vi "AlarmasGlobal.vi"() -> ()   [LabVIEW 2018]
uses:
  Controls/Cluster_Alarmas_IEEE45.ctl
  <vilib>/RAFA Solutions/Harmony UI Controls Kit/Boolean/Round Led.ctl
  <vilib>/RAFA Solutions/Harmony UI Controls Kit/Flat UI Design.lvlib
panel:
  out "G06_Alarmas_IEEE45":T1={"V1_V2 (V) "={0.0, 17.0, 16.662651515468255}, "Mod_V1_V2"=0.0, "alarma 1"=FALSE, "Mod_V2_V3"=0.0, "alarma 2"=FALSE, "Mod_V3_V1"=0.0, "alarma 3"=FALSE, "Mod_Frec"=0.0, "alarma 4"=FALSE, "V2_V3 (V)"={0.0, 17.0, 16.662651515468255}, "V3_V1 (V)"={0.0, 17.0, 16.662651515468255}, "Frecuencia (Hz)"={0.0, 17.0, 16.662651515468255}, "AVG VL_VL (V)"={0.0, 17.0, 16.662651515468255}, "alarm 5"=FALSE, "alarm 6"=FALSE, "alarm 7"=FALSE, "alarm 8"=FALSE, "alarm 9"=FALSE} {"AVG VL_VL (V)" scale=427.0..473.0; "Frecuencia (Hz)" scale=58.0..62.0; "V3_V1 (V)" scale=418.0..482.0; "V2_V3 (V)" scale=418.0..482.0; "Mod_Frec" format="%#.1f"; "Mod_V3_V1" format="%#.1f"; "Mod_V2_V3" format="%#.1f"; "Mod_V1_V2" format="%#.1f"; "V1_V2 (V)" scale=418.0..482.0}
  out "G05_Alarmas_IEEE45":T1={"V1_V2 (V) "={0.0, 17.0, 16.662651515468255}, "Mod_V1_V2"=0.0, "alarma 1"=FALSE, "Mod_V2_V3"=0.0, "alarma 2"=FALSE, "Mod_V3_V1"=0.0, "alarma 3"=FALSE, "Mod_Frec"=0.0, "alarma 4"=FALSE, "V2_V3 (V)"={0.0, 17.0, 16.662651515468255}, "V3_V1 (V)"={0.0, 17.0, 16.662651515468255}, "Frecuencia (Hz)"={0.0, 17.0, 16.662651515468255}, "AVG VL_VL (V)"={0.0, 17.0, 16.662651515468255}, "alarm 5"=FALSE, "alarm 6"=FALSE, "alarm 7"=FALSE, "alarm 8"=FALSE, "alarm 9"=FALSE} {"AVG VL_VL (V)" scale=427.0..473.0; "Frecuencia (Hz)" scale=58.0..62.0; "V3_V1 (V)" scale=418.0..482.0; "V2_V3 (V)" scale=418.0..482.0; "Mod_Frec" format="%#.1f"; "Mod_V3_V1" format="%#.1f"; "Mod_V2_V3" format="%#.1f"; "Mod_V1_V2" format="%#.1f"; "V1_V2 (V)" scale=418.0..482.0}
  out "G04_Alarmas_IEEE45":T1={"V1_V2 (V) "={0.0, 17.0, 16.662651515468255}, "Mod_V1_V2"=0.0, "alarma 1"=FALSE, "Mod_V2_V3"=0.0, "alarma 2"=FALSE, "Mod_V3_V1"=0.0, "alarma 3"=FALSE, "Mod_Frec"=0.0, "alarma 4"=FALSE, "V2_V3 (V)"={0.0, 17.0, 16.662651515468255}, "V3_V1 (V)"={0.0, 17.0, 16.662651515468255}, "Frecuencia (Hz)"={0.0, 17.0, 16.662651515468255}, "AVG VL_VL (V)"={0.0, 17.0, 16.662651515468255}, "alarm 5"=FALSE, "alarm 6"=FALSE, "alarm 7"=FALSE, "alarm 8"=FALSE, "alarm 9"=FALSE} {"AVG VL_VL (V)" scale=427.0..473.0; "Frecuencia (Hz)" scale=58.0..62.0; "V3_V1 (V)" scale=418.0..482.0; "V2_V3 (V)" scale=418.0..482.0; "Mod_Frec" format="%#.1f"; "Mod_V3_V1" format="%#.1f"; "Mod_V2_V3" format="%#.1f"; "Mod_V1_V2" format="%#.1f"; "V1_V2 (V)" scale=418.0..482.0}
  out "G03_Alarmas_IEEE45":T1={"V1_V2 (V) "={0.0, 17.0, 16.662651515468255}, "Mod_V1_V2"=0.0, "alarma 1"=FALSE, "Mod_V2_V3"=0.0, "alarma 2"=FALSE, "Mod_V3_V1"=0.0, "alarma 3"=FALSE, "Mod_Frec"=0.0, "alarma 4"=FALSE, "V2_V3 (V)"={0.0, 17.0, 16.662651515468255}, "V3_V1 (V)"={0.0, 17.0, 16.662651515468255}, "Frecuencia (Hz)"={0.0, 17.0, 16.662651515468255}, "AVG VL_VL (V)"={0.0, 17.0, 16.662651515468255}, "alarm 5"=FALSE, "alarm 6"=FALSE, "alarm 7"=FALSE, "alarm 8"=FALSE, "alarm 9"=FALSE} {"AVG VL_VL (V)" scale=427.0..473.0; "Frecuencia (Hz)" scale=58.0..62.0; "V3_V1 (V)" scale=418.0..482.0; "V2_V3 (V)" scale=418.0..482.0; "Mod_Frec" format="%#.1f"; "Mod_V3_V1" format="%#.1f"; "Mod_V2_V3" format="%#.1f"; "Mod_V1_V2" format="%#.1f"; "V1_V2 (V)" scale=418.0..482.0}
  out "G02_Alarmas_IEEE45":T1={"V1_V2 (V) "={0.0, 17.0, 16.662651515468255}, "Mod_V1_V2"=0.0, "alarma 1"=FALSE, "Mod_V2_V3"=0.0, "alarma 2"=FALSE, "Mod_V3_V1"=0.0, "alarma 3"=FALSE, "Mod_Frec"=0.0, "alarma 4"=FALSE, "V2_V3 (V)"={0.0, 17.0, 16.662651515468255}, "V3_V1 (V)"={0.0, 17.0, 16.662651515468255}, "Frecuencia (Hz)"={0.0, 17.0, 16.662651515468255}, "AVG VL_VL (V)"={0.0, 17.0, 16.662651515468255}, "alarm 5"=FALSE, "alarm 6"=FALSE, "alarm 7"=FALSE, "alarm 8"=FALSE, "alarm 9"=FALSE} {"AVG VL_VL (V)" scale=427.0..473.0; "Frecuencia (Hz)" scale=58.0..62.0; "V3_V1 (V)" scale=418.0..482.0; "V2_V3 (V)" scale=418.0..482.0; "Mod_Frec" format="%#.1f"; "Mod_V3_V1" format="%#.1f"; "Mod_V2_V3" format="%#.1f"; "Mod_V1_V2" format="%#.1f"; "V1_V2 (V)" scale=418.0..482.0}
  out "G01_Alarmas_IEEE45":T1={"V1_V2 (V) "={0.0, 17.0, 16.662651515468255}, "Mod_V1_V2"=0.0, "alarma 1"=FALSE, "Mod_V2_V3"=0.0, "alarma 2"=FALSE, "Mod_V3_V1"=0.0, "alarma 3"=FALSE, "Mod_Frec"=0.0, "alarma 4"=FALSE, "V2_V3 (V)"={0.0, 17.0, 16.662651515468255}, "V3_V1 (V)"={0.0, 17.0, 16.662651515468255}, "Frecuencia (Hz)"={0.0, 17.0, 16.662651515468255}, "AVG VL_VL (V)"={0.0, 17.0, 16.662651515468255}, "alarm 5"=FALSE, "alarm 6"=FALSE, "alarm 7"=FALSE, "alarm 8"=FALSE, "alarm 9"=FALSE} {"AVG VL_VL (V)" scale=427.0..473.0; "Frecuencia (Hz)" scale=58.0..62.0; "V3_V1 (V)" scale=418.0..482.0; "V2_V3 (V)" scale=418.0..482.0; "Mod_Frec" format="%#.1f"; "Mod_V3_V1" format="%#.1f"; "Mod_V2_V3" format="%#.1f"; "Mod_V1_V2" format="%#.1f"; "V1_V2 (V)" scale=418.0..482.0}
  # "Tolerancias"
  # "Modulación"
  # "%"
  # "%"
  # "%"
  # "5 % máx."
  # "%"
  # "0,5 % máx."
  # "Tolerancias"
  # "Modulación"
  # "%"
  # "%"
  # "%"
  # "5 % máx."
  # "%"
  # "0,5 % máx."
  # "Tolerancias"
  # "Modulación"
  # "%"
  # "%"
  # "%"
  # "5 % máx."
  # "%"
  # "0,5 % máx."
  # "Tolerancias"
  # "Modulación"
  # "%"
  # "%"
  # "%"
  # "5 % máx."
  # "%"
  # "0,5 % máx."
  # "Tolerancias"
  # "Modulación"
  # "%"
  # "%"
  # "%"
  # "5 % máx."
  # "%"
  # "0,5 % máx."
  # "Tolerancias"
  # "Modulación"
  # "%"
  # "%"
  # "%"
  # "5 % máx."
  # "%"
  # "0,5 % máx."
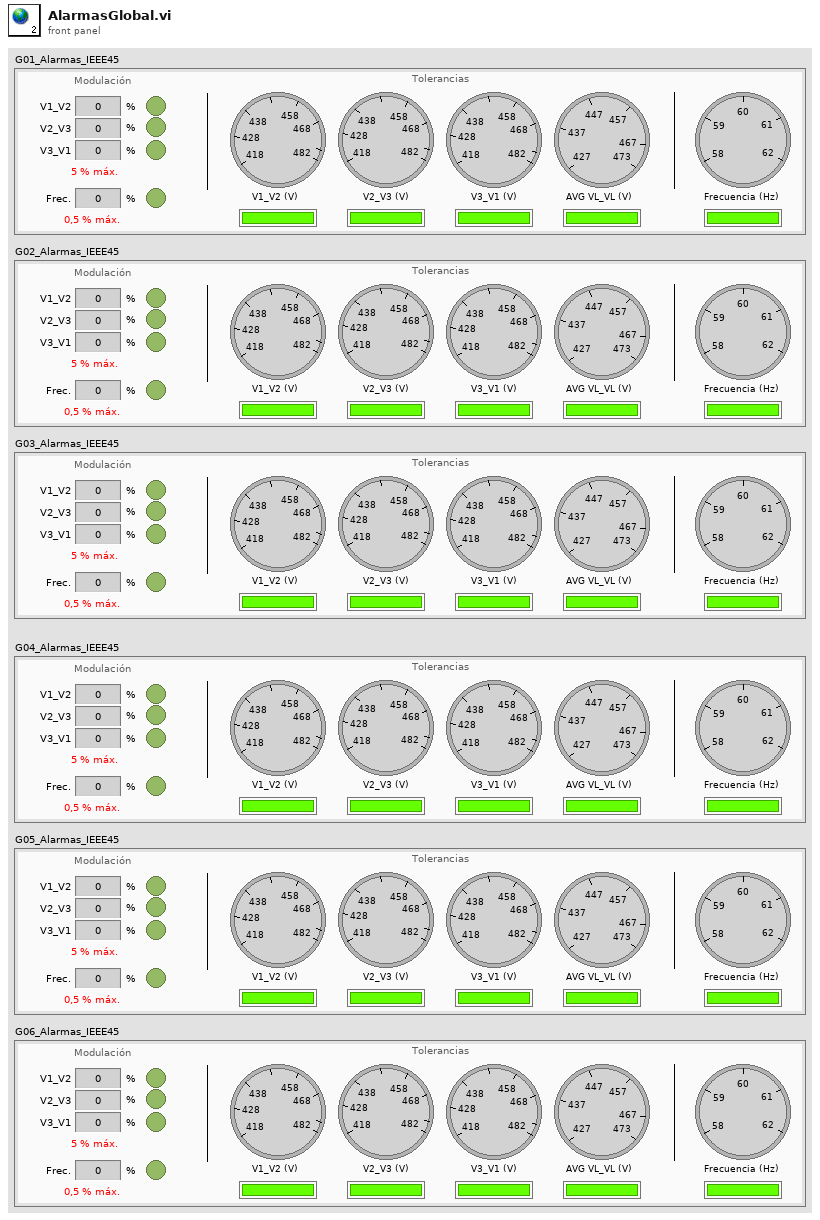
[diagram p1: front panel]
types:
  T1 = typedef "Cluster_Alarmas_IEEE45.ctl" = cluster{"V1_V2 (V) ":cluster{dbl, dbl, dbl}, "Mod_V1_V2":dbl, "alarma 1":T2, "Mod_V2_V3":dbl, "alarma 2":T2, "Mod_V3_V1":dbl, "alarma 3":T2, "Mod_Frec":dbl, "alarma 4":T2, "V2_V3 (V)":cluster{dbl, dbl, dbl}, "V3_V1 (V)":cluster{dbl, dbl, dbl}, "Frecuencia (Hz)":cluster{dbl, dbl, dbl}, "AVG VL_VL (V)":cluster{dbl, dbl, dbl}, "alarm 5":bool, "alarm 6":bool, "alarm 7":bool, "alarm 8":bool, "alarm 9":bool}
  T2 = typedef "Flat UI Design.lvlib/Round Led.ctl" = bool
diagram:
